vi "create available tags menu.vi"(8 "error in":errorcluster, 9 "channel to map to":refnum<class "TBM channel.lvclass">, 10 "MenuRef":refnum<k9>, 11 "engine configuration in":refnum<class "engine configuration.lvclass">) -> (0 "error out":errorcluster, 3 "engine configuration out":refnum<class "engine configuration.lvclass">)   [LabVIEW 2013, in "fixed channel editor.lvclass"]
uses:
  fixed channel editor.lvclass
  <vilib>/NI/Module Execution Interface/Engine Configuration/engine configuration.lvclass
  <vilib>/NI/Tag Bus Module Framework/channel/TBM channel.lvclass
  <vilib>/NI/Tag Bus/tag/tag descriptor.lvclass/tag descriptor.ctl
  <vilib>/NI/Tag Bus/tag/read tag name.vi
  <vilib>/NI/Tag Bus/tag/tag descriptor.lvclass
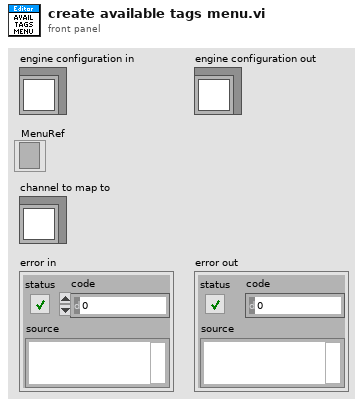
[diagram p1: front panel]
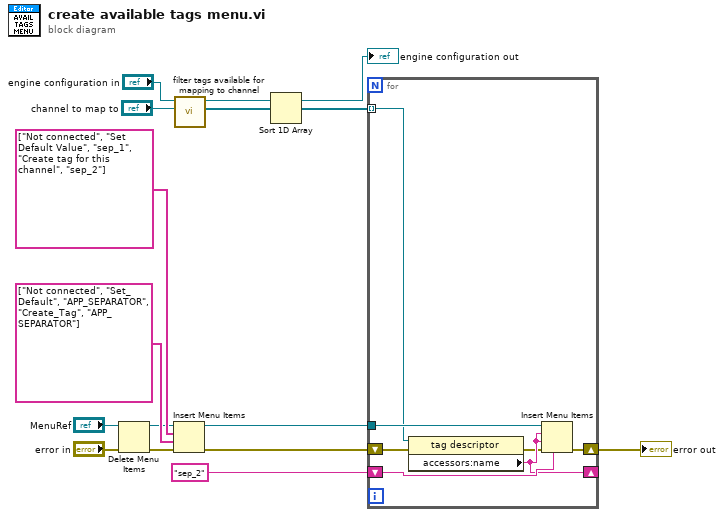
[diagram p0: block diagram]
diagram:
  n1 = Delete Menu Items(6:"error in", 9:"MenuRef") -> (0:w3:errorcluster, 3:w4:refnum<k9>)  [unwired: 2 in]
  n2 = Insert Menu Items(6:w3, 7:string[] ["Not connected", "Set_Default", "APP_SEPARATOR", "Create_Tag", "APP_SEPARATOR"] ("item tags"), 8:string[] ["Not connected", "Set Default Value", "sep_1", "Create tag for this channel", "sep_2"] ("item names"), 9:w4) -> (0:w8:errorcluster, 3:w11:refnum<k9>)  [unwired: 2 in, 1 out]
  n3 = call <vilib>:"filter tags available for mapping to channel.vi"("channel to map to"="channel to map to", "engine configuration in"="engine configuration in") -> ("filtered tags"=w10:refnum<class "tag descriptor.lvclass">[], "engine configuration out"=→"engine configuration out":refnum<class "engine configuration.lvclass">)  [unwired: 8 in]
  n4 = Sort 1D Array(array=w10) -> (sorted array=w1:refnum<class "tag descriptor.lvclass">[])
  n5 = for {
    tunnel: w11 -> [w22]
    tunnel: w1 -> [w21] mode=indexing
    shift-right: [w19] -> _
    shift-left: "sep_2" -> [w20]
    shift-right: [w16] -> w7
    shift-left: w8 -> [w18]
    n6 = property class="tag descriptor"(reference=w21, error in=w18) -> (error out=w17:errorcluster, "accessors:name"=w19:string)  [unwired: 1 out]
    n7 = Insert Menu Items(4:w20, 6:w17, 7:w19, 8:w19, 9:w22) -> (0:w16:errorcluster)  [unwired: 1 in, 2 out]
  }
  "error out" <- w7
